vi "Syringe_getSize.vi"(11 "Ring Refnum":refnum<vi>) -> (1 "Syringe Size":dbl, 2 "StandardSize":bool, 3 "Syringe Area":dbl)   [LabVIEW 2015]
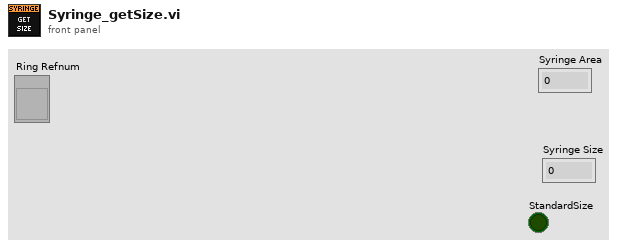
[diagram p1: front panel]
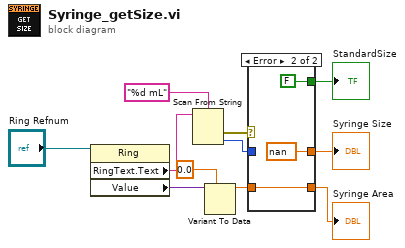
[diagram p0: block diagram]
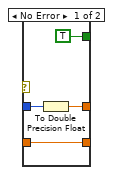
[diagram p2: hidden frame]
diagram:
  n1 = property class="Ring"(reference="Ring Refnum") -> ("RingText.Text"=w6:string, "Value"=w4:variant)  [unwired: 1 in, 2 out]
  n2 = Scan From String(format string="%d mL", input string=w6) -> (error out=w10:errorcluster, output 1=w9:i32)  [unwired: 3 in, 2 out]
  n3 = Variant To Data(type=0.0, Variant=w4) -> (data=w2:dbl)  [unwired: 1 in, 1 out]
  n4 = case shown="Error" w10 {
    tunnel: w9 -> [w13 _]
    tunnel: [w14 w17] -> w8
    tunnel: [TRUE FALSE] -> w7
    tunnel: w2 -> [w14 w17]
    tunnel: [w12 nan] -> w1
    frame No Error {
      n5 = To Double Precision Float(number=w13) -> (double precision float=w12:dbl)
    }
    frame Error {
    }
  }
  "Syringe Area" <- w8
  "StandardSize" <- w7
  "Syringe Size" <- w1
